vi "helloworld.vi"() -> ()   [LabVIEW 2020]
panel:
  in  "index":i32
  out "element":dbl
  out "size(s)":i32
  out "Array 2":u8[](array[slide]) scale=0.0..100.0
  in  "Array":dbl[](array[numeric])
  out "Waveform Graph":dbl[](graph)
  out "Numeric 3":dbl
  out "Waveform Chart":dbl(graph)
  in  "stop":bool
  in  "Slide 8":dbl(slide) scale=0.0..200.0
  in  "Slide 7":dbl(slide) scale=0.0..10.0
  in  "Slide 6":dbl(slide) scale=0.0..10.0
  in  "Slide 5":dbl(slide) scale=0.0..10.0
  out "Meter":dbl(knob) scale=0.0..10.0
  out "Tank":dbl(slide) scale=0.0..10.0
  out "Thermometer":dbl(slide) scale=0.0..10.0
  out "Slide 4":u8(slide) scale=0.0..100.0 scale format="%.5f"
  out "Slide 3":u8(slide) scale=0.0..100.0
  in  "Slide 2":dbl(slide) scale=0.0..100.0
  in  "Slide":dbl(slide) scale=0.0..78.0
  out "Time Stamp 2":timestamp
  in  "Time Stamp":timestamp
  out "Numeric 2":dbl
  in  "Numeric":dbl
  out "String":string caption="Output"
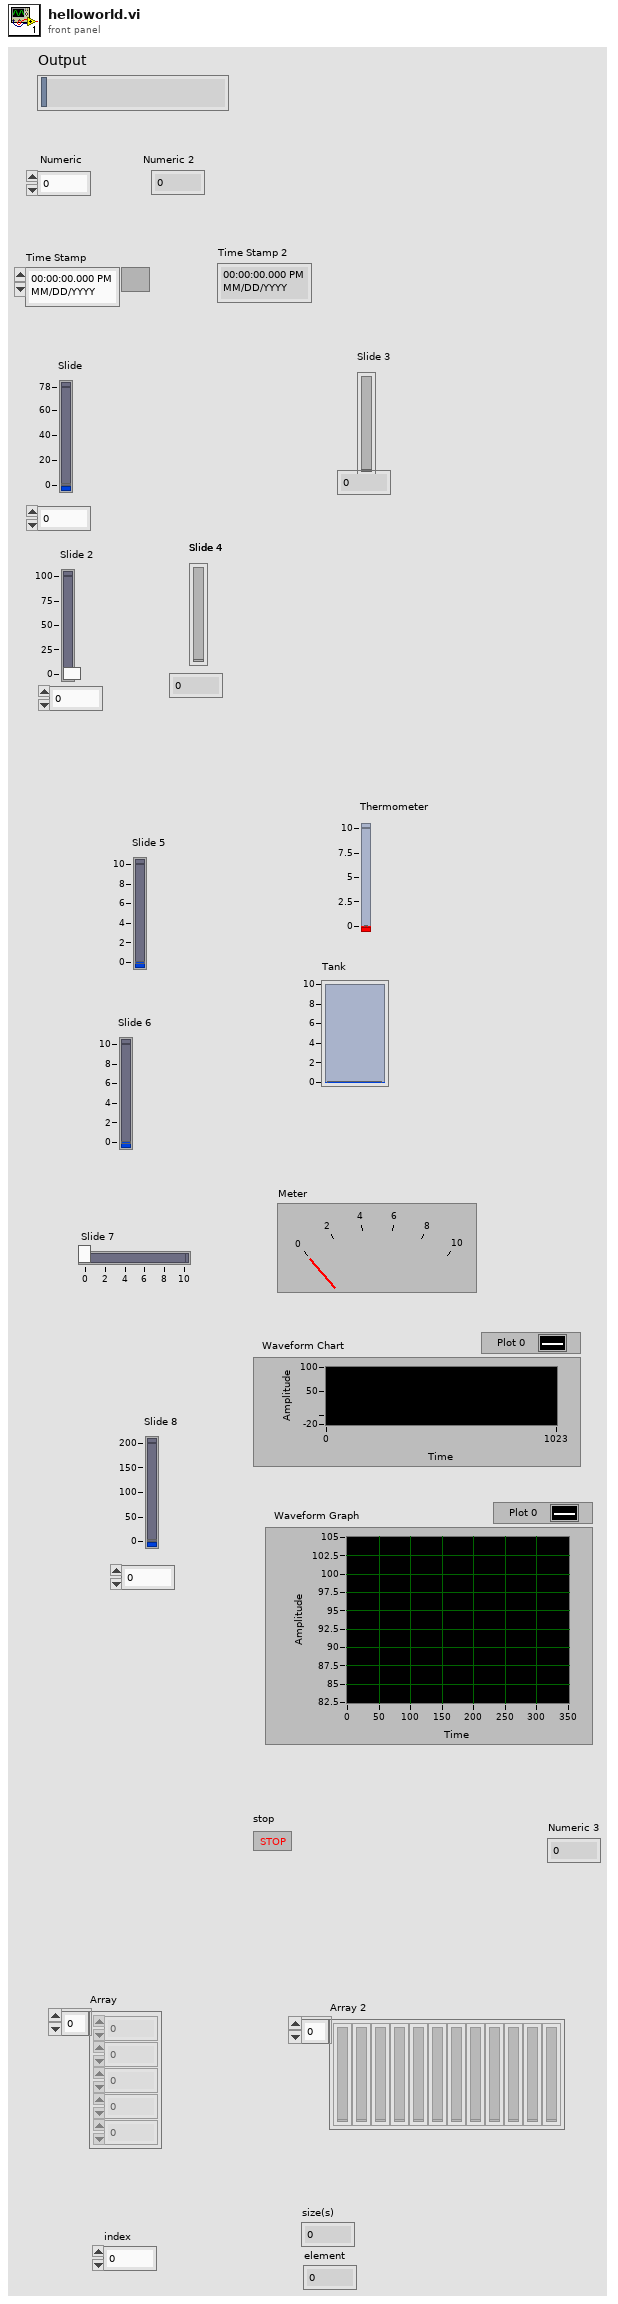
[diagram p1: front panel]
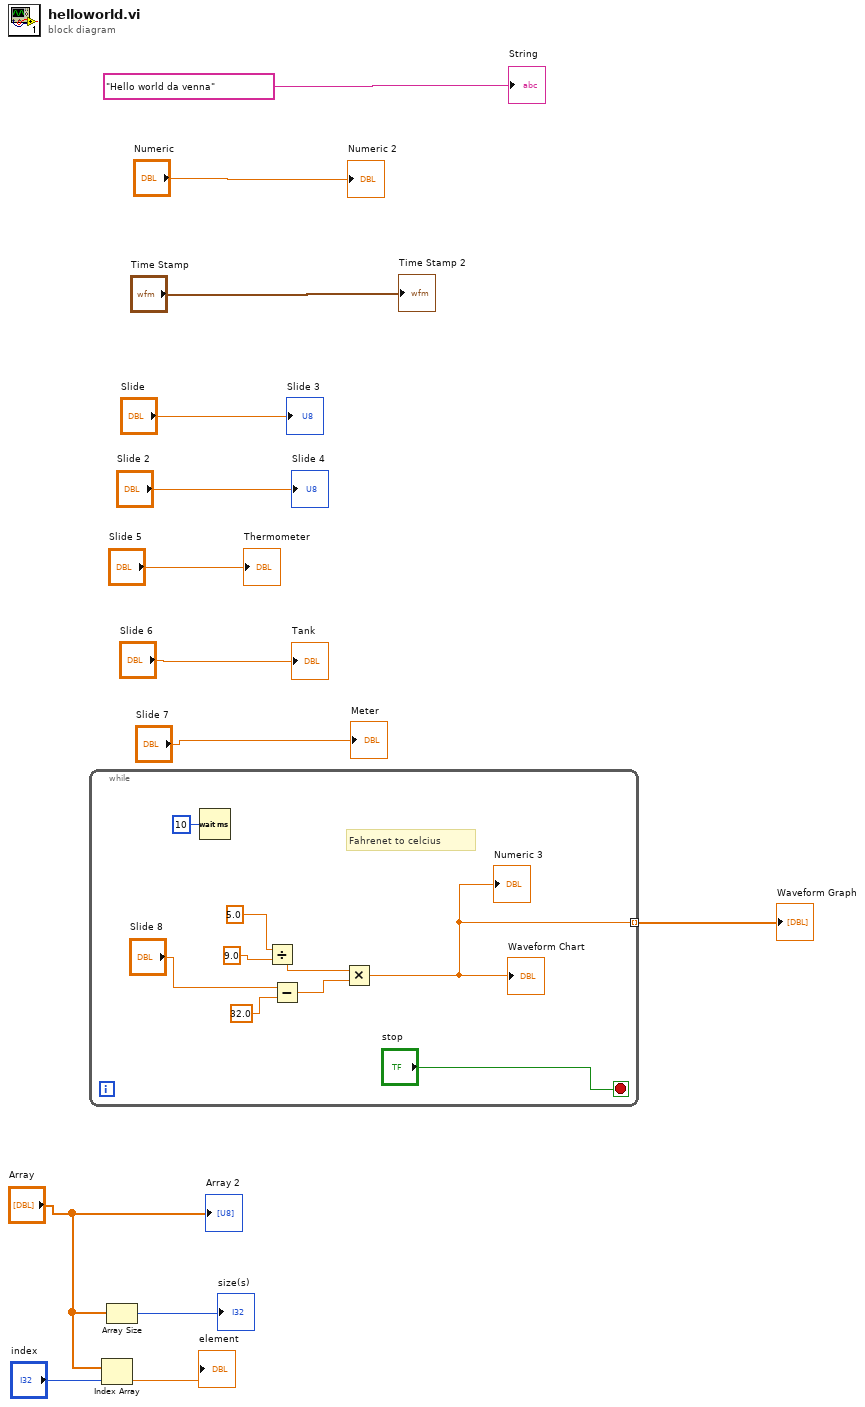
[diagram p0: block diagram]
diagram:
  n1 = while {
    tunnel: [w14] -> w5 mode=indexing
    stop <- "stop" stop-if-true
    # "Fahrenet to celcius"
    n2 = Wait (ms)(milliseconds to wait=u32 10) -> ()  [unwired: 1 out]
    n3 = Divide(x=5.0, y=9.0) -> (x/y=w20:dbl)
    n4 = Subtract(x="Slide 8", y=32.0) -> (x-y=w21:dbl)
    n5 = Multiply(x=w20, y=w21) -> (x*y=w14:dbl)
    "Waveform Chart" <- w14
    "Numeric 3" <- w14
  }
  "Waveform Graph" <- w5
  n6 = Index Array(array="Array", index="index") -> (element=→"element":dbl)
  n7 = Array Size(array="Array") -> (size(s)=→"size(s)":i32)
  "String" <- "Hello world da venna"
  "Numeric 2" <- "Numeric"
  "Time Stamp 2" <- "Time Stamp"
  "Slide 3" <- "Slide"
  "Slide 4" <- "Slide 2"
  "Thermometer" <- "Slide 5"
  "Tank" <- "Slide 6"
  "Meter" <- "Slide 7"
  "Array 2" <- "Array"
